vi "File_Name_Append_Suffix.vi"(7 "Suffix":string, 11 "Path":path) -> (3 "appended path":path)   [LabVIEW 2020]
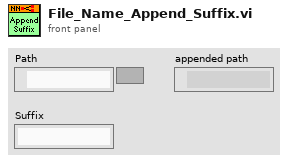
[diagram p1: front panel]
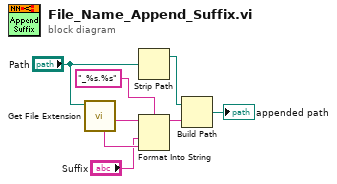
[diagram p0: block diagram]
diagram:
  n1 = call <vilib>:"Get File Extension.vi"("file"="Path") -> ("filename without extension"=w2:string, "unmodified file extension"=w5:string)  [unwired: 6 in, 3 out]
  n2 = Strip Path(path="Path") -> (stripped path=w6:path)  [unwired: 1 out]
  n3 = Format Into String(format string="_%s.%s", initial string=w2, "Suffix", w5) -> (resulting string=w7:string)  [unwired: 1 in, 1 out]
  n4 = Build Path(base path=w6, name or relative path=w7) -> (appended path=→"appended path":path)
